vi "Auto Drive Y.vi"(0 "PID Gains":T1={"proportional gain (Kc)"=0.07, "integral time (Ti, min)"=0.0, "derivative time (Td, min)"=0.0}, 4 "Max Time (ms)":u32=15000, 6 "Min Time (ms)":u32=250, 8 "Time to Settle (ms)":u32=50, 9 "Distance (in)":dbl=15.0 format="%#_13g", 10 "Motor Output Range":cluster{"output high":dbl, "output low":dbl}={"output high"=0.7, "output low"=-0.7}, 11 "RobotDriveDevRef In":T2={"DevStatus"={"status"=FALSE, "code"=0, "source"=""}, "Motors[]"=[], "Square Inputs"=FALSE, "Max Output"=1.0}) -> (3 "RobotDriveDevRef Out":T2={"DevStatus"={"status"=FALSE, "code"=0, "source"=""}, "Motors[]"=[], "Square Inputs"=FALSE, "Max Output"=1.0})   [LabVIEW 2017]
uses:
  <vilib>/Rock Robotics/WPI/RobotDrive/WPI_RobotDriveDevRef.ctl
  <vilib>/Rock Robotics/WPI/MotorControl/WPI_MotorControlDeviceRef.ctl
  <vilib>/Rock Robotics/WPI/MotorControl/WPI_MotorControlType.ctl
  <vilib>/Rock Robotics/SystemInterfaces/DIO/FPGA_DIOPWMChannel.ctl
  <vilib>/Rock Robotics/WPI/PWM/WPI_PWMDeadband.ctl
  <vilib>/Rock Robotics/SystemInterfaces/DIO/FPGA_DIOChannel.ctl
  Globals/Robot Global Data.vi
  <vilib>/addons/control/pid/pid.llb/PID (DBL).vi
  <vilib>/Rock Robotics/WPI/RobotDrive/WPI_RobotDriveArcadeDrive_Standard(NoSaturation).vi
  <vilib>/addons/control/pid/NI_PID_pid.lvlib
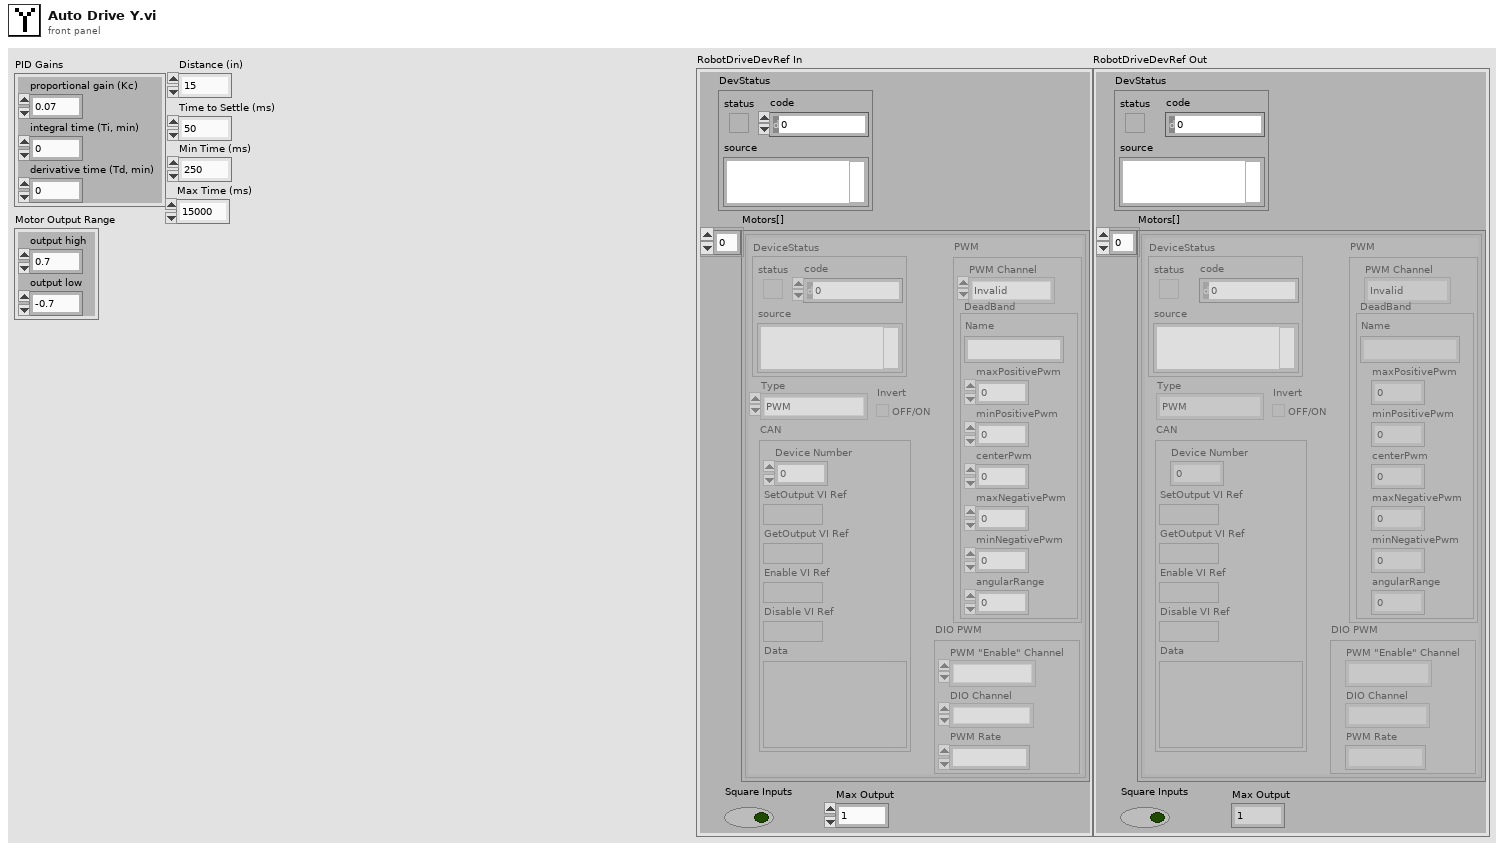
[diagram p1: front panel]
types:
  T1 = cluster{"proportional gain (Kc)":dbl, "integral time (Ti, min)":dbl, "derivative time (Td, min)":dbl}
  T2 = typedef "WPI_RobotDriveDevRef.ctl" = cluster{"DevStatus":errorcluster, "Motors[]":T3[], "Square Inputs":bool, "Max Output":dbl}
  T3 = typedef "WPI_MotorControlDeviceRef.ctl" = cluster{"DeviceStatus":errorcluster, "Type":T4, "PWM":cluster{"PWM Channel":T5, "DeadBand":T6}, "CAN":cluster{"Device Number":u8, "SetOutput VI Ref":variant, "GetOutput VI Ref":variant, "Enable VI Ref":variant, "Disable VI Ref":variant, "Data":variant}, "Invert":bool, "DIO PWM":cluster{"PWM \"Enable\" Channel":T5, "DIOChannel":T7, "PWM Rate":dbl}}
  T4 = typedef "WPI_MotorControlType.ctl" = enum16{"PWM", "CAN", "DIO PWM"}
  T5 = typedef "FPGA_DIOPWMChannel.ctl" = enum8{"PWM 0", "PWM 1", "PWM 2", "PWM 3", "PWM 4", "PWM 5", "PWM 6", "PWM 7", "PWM 8", "PWM 9", "PWM MXP 0", "PWM MXP 1", "PWM MXP 2", "PWM MXP 3", "PWM MXP 4", "PWM MXP 5", "PWM MXP 6", "PWM MXP 7", "PWM MXP 8", "PWM MXP 9", "Invalid"}
  T6 = typedef "WPI_PWMDeadband.ctl" = cluster{"Name":string, "maxPositivePwm":i32, "minPositivePwm":i32, "centerPwm":i32, "maxNegativePwm":i32, "minNegativePwm":i32, "angularRange":u16}
  T7 = typedef "FPGA_DIOChannel.ctl" = enum8{"DIO 0", "DIO 1", "DIO 2", "DIO 3", "DIO 4", "DIO 5", "DIO 6", "DIO 7", "DIO 8", "DIO 9", "DIO MXP 0", "DIO MXP 1", "DIO MXP 2", "DIO MXP 3", "DIO MXP 4", "DIO MXP 5", "DIO MXP 6", "DIO MXP 7", "DIO MXP 8", "DIO MXP 9", "DIO MXP 10", "DIO MXP 11", "DIO MXP 12", "DIO MXP 13", "DIO MXP 14", "DIO MXP 15", "SPI Port CS1", "SPI Port CS2", "SPI Port CS3", "SPI Port MISO", "SPI Port MOSI", "Invalid"}
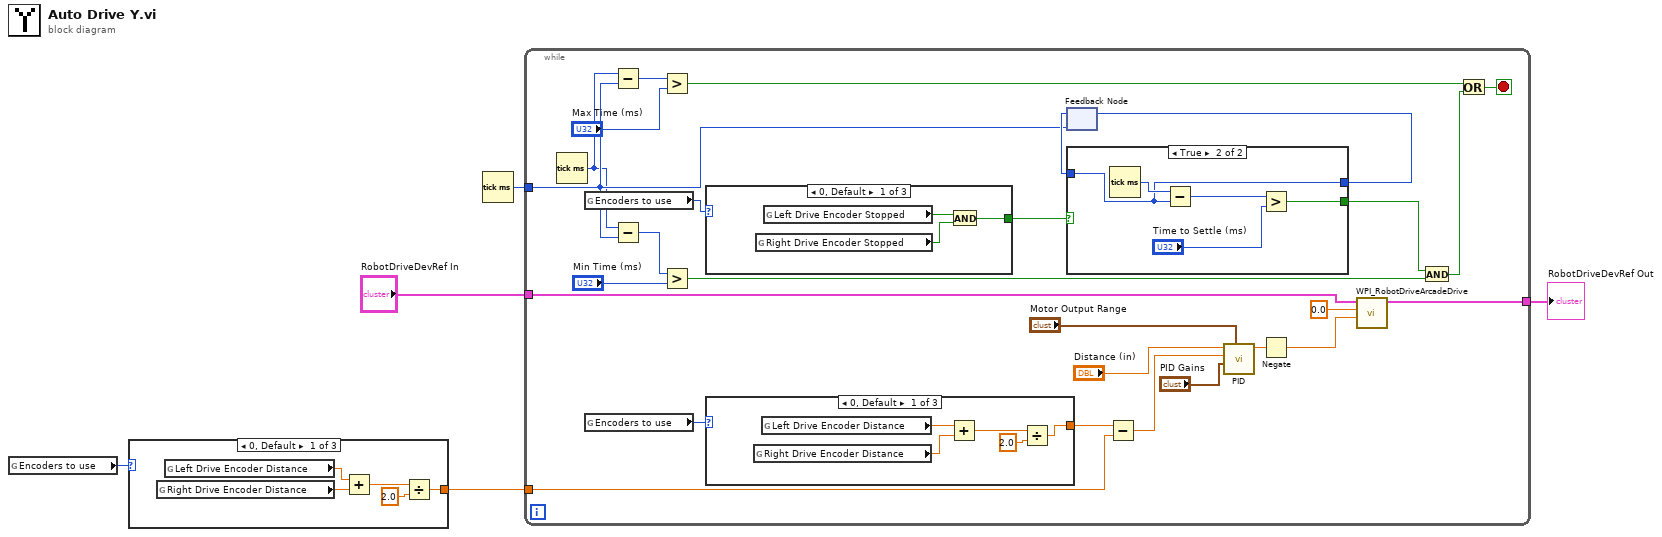
[diagram p0: block diagram]
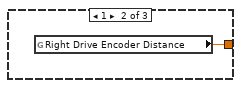
[diagram p2: hidden frame]
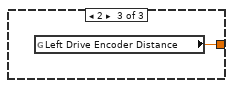
[diagram p3: hidden frame]
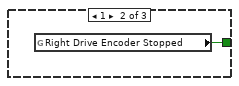
[diagram p4: hidden frame]
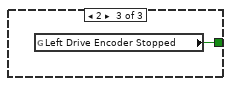
[diagram p5: hidden frame]
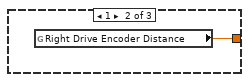
[diagram p6: hidden frame]
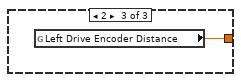
[diagram p7: hidden frame]
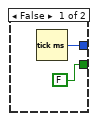
[diagram p8: hidden frame]
diagram:
  n1 = global read "Robot Global Data.vi" "Encoders to use"() -> (w1:u16)
  n2 = case shown="0, Default" w1 {
    tunnel: [w6 w11 w12] -> w5
    frame 0, Default {
      n3 = global read "Robot Global Data.vi" "Right Drive Encoder Distance"() -> (w9:dbl)
      n4 = global read "Robot Global Data.vi" "Left Drive Encoder Distance"() -> (w10:dbl)
      n5 = Add(x=w10, y=w9) -> (x+y=w8:dbl)
      n6 = Divide(x=w8, y=2.0) -> (x/y=w6:dbl)
    }
    frame 1 {
      n7 = global read "Robot Global Data.vi" "Right Drive Encoder Distance"() -> (w11:dbl)
    }
    frame 2 {
      n8 = global read "Robot Global Data.vi" "Left Drive Encoder Distance"() -> (w12:dbl)
    }
  }
  n9 = Tick Count (ms)() -> (millisecond timer value=w4:u32)
  n10 = while {
    tunnel: "RobotDriveDevRef In" -> [w36]
    tunnel: w5 -> [w30]
    tunnel: w4 -> [w18]
    tunnel: [w28] -> w3
    stop <- w21 stop-if-true
    n11 = Tick Count (ms)() -> (millisecond timer value=w17:u32)
    n12 = global read "Robot Global Data.vi" "Encoders to use"() -> (w14:u16)
    n13 = global read "Robot Global Data.vi" "Encoders to use"() -> (w16:u16)
    n14 = Subtract(x=w17, y=w18) -> (x-y=w22:u32)
    n15 = Subtract(x=w17, y=w18) -> (x-y=w27:u32)
    n16 = Greater?(x=w22, y="Max Time (ms)") -> (0:w19:bool)
    n17 = Greater?(x=w27, y="Min Time (ms)") -> (0:w24:bool)
    n18 = case shown="0, Default" w14 {
      tunnel: [w42 w43 w44] -> w13
      frame 0, Default {
        n19 = global read "Robot Global Data.vi" "Right Drive Encoder Stopped"() -> (w40:bool)
        n20 = global read "Robot Global Data.vi" "Left Drive Encoder Stopped"() -> (w41:bool)
        n21 = And(x=w41, y=w40) -> (x .and. y?=w42:bool)
      }
      frame 1 {
        n22 = global read "Robot Global Data.vi" "Right Drive Encoder Stopped"() -> (w43:bool)
      }
      frame 2 {
        n23 = global read "Robot Global Data.vi" "Left Drive Encoder Stopped"() -> (w44:bool)
      }
    }
    n24 = case shown="0, Default" w16 {
      tunnel: [w45 w50 w51] -> w15
      frame 0, Default {
        n25 = global read "Robot Global Data.vi" "Right Drive Encoder Distance"() -> (w48:dbl)
        n26 = global read "Robot Global Data.vi" "Left Drive Encoder Distance"() -> (w49:dbl)
        n27 = Add(x=w49, y=w48) -> (x+y=w47:dbl)
        n28 = Divide(x=w47, y=2.0) -> (x/y=w45:dbl)
      }
      frame 1 {
        n29 = global read "Robot Global Data.vi" "Right Drive Encoder Distance"() -> (w50:dbl)
      }
      frame 2 {
        n30 = global read "Robot Global Data.vi" "Left Drive Encoder Distance"() -> (w51:dbl)
      }
    }
    n31 = feedback #1(w18) -> (w31:u32)
    n32 = case shown="True" w13 {
      tunnel: w31 -> [_ w57]
      tunnel: [w53 w57] -> w32
      tunnel: [FALSE w54] -> w25
      frame False {
        n33 = Tick Count (ms)() -> (millisecond timer value=w53:u32)
      }
      frame True {
        n34 = Tick Count (ms)() -> (millisecond timer value=w58:u32)
        n35 = Subtract(x=w58, y=w57) -> (x-y=w56:u32)
        n36 = Greater?(x=w56, y="Time to Settle (ms)") -> (0:w54:bool)
      }
    }
    n37 = feedback-in #1(w32) -> ()
    n38 = Subtract(x=w15, y=w30) -> (x-y=w29:dbl)
    n39 = call-poly <vilib>:"PID.vi"("output range"="Motor Output Range", "PID gains"="PID Gains", "process variable"=w29, "setpoint"="Distance (in)") -> ("output"=w33:dbl)  [unwired: 6 in, 1 out]
    n40 = Negate(x=w33) -> (-x=w34:dbl)
    n41 = call-poly <vilib>:"WPI_RobotDriveArcadeDrive.vi"("Y axis value"=w34, "X axis value"=0.0, "RobotDriveDevRef"=w36) -> ("RobotDriveDevRef"=w28:T2)  [unwired: 6 in, 2 out]
    n42 = And(x=w25, y=w24) -> (x .and. y?=w20:bool)
    n43 = Or(x=w19, y=w20) -> (x .or. y?=w21:bool)
  }
  "RobotDriveDevRef Out" <- w3
